vi "DK240 SlitAdjust.vi"(4 "Fente":enum16{"Entrée", "Sortie"}(ring), 5 "error in":errorcluster, 6 "SlitWidth":u16=50 caption="Largeur \nFente (µm)" max=5000 step=1, 7 "MovingRef":refnum<vi>, 8 "Port":refnum<visa-resource-name>="SPECTRO") -> (0 "error out":errorcluster, 2 "Moving":bool caption="Déplacement\nen cours", 3 "Status":u8)   [LabVIEW 2019]
doc: "Ce Vi ajuste la largeur de la fente spécifié à la valeur, en microns, désirée."
uses:
  <vilib>/Utility/error.llb/DialogType.ctl
panel:
  out "Cancel":u8
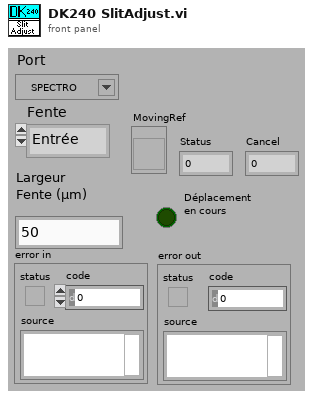
[diagram p1: front panel]
types:
  T1 = enum16{"Commande", "AttendPrêt", "Paramètre", "AttendFin", "Statut", "Fin"}
  T2 = typedef "DialogType.ctl" = u16
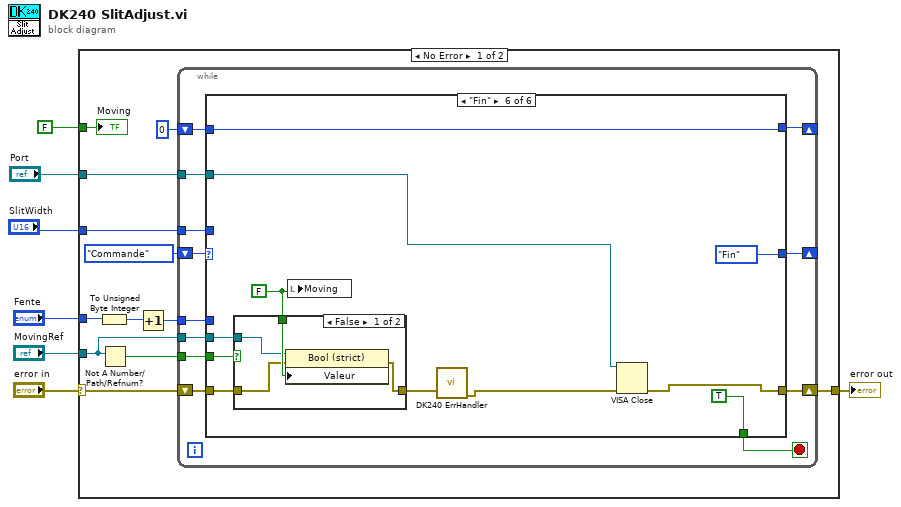
[diagram p0: block diagram]
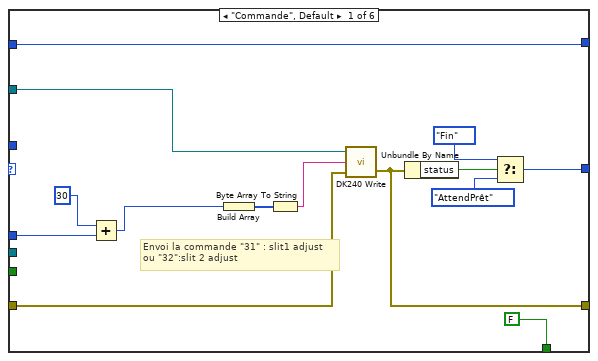
[diagram p2: hidden frame]
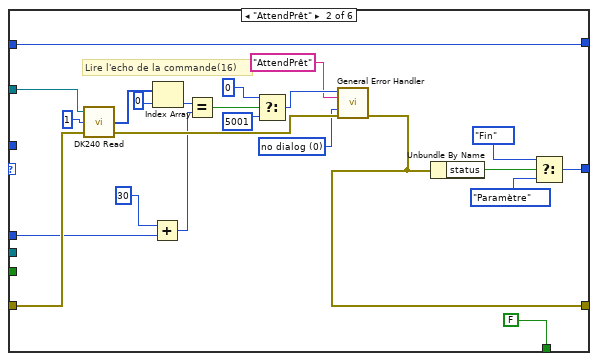
[diagram p3: hidden frame]
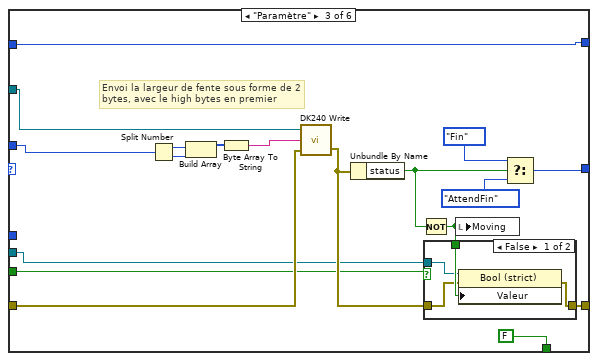
[diagram p4: hidden frame]
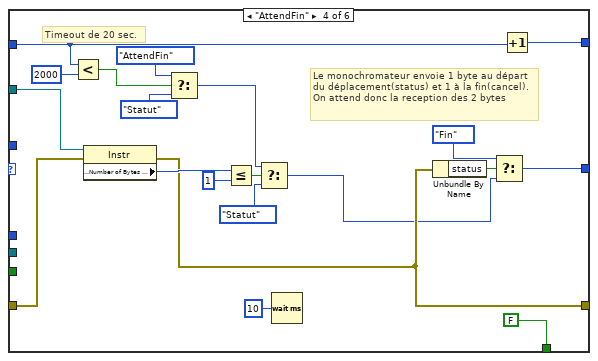
[diagram p6: hidden frame]
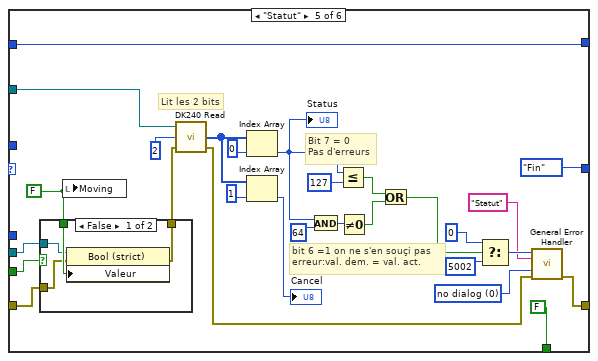
[diagram p7: hidden frame]
diagram:
  n1 = case shown="No Error" "error in" {
    selector: "error in" -> [w15 w161]
    tunnel: "Port" -> [w18 _]
    tunnel: "SlitWidth" -> [w17 _]
    tunnel: [w16 w161] -> w6
    tunnel: FALSE ("Moving") -> [w14 _]
    tunnel: "Fente" -> [w9 _]
    tunnel: "MovingRef" -> [w10 _]
    frame No Error {
      n2 = To Unsigned Byte Integer(number=w9) -> (unsigned 8bit integer=w8:u8)
      n3 = Not A Number/Path/Refnum?(number/path/refnum=w10) -> (NaN/Path/Refnum?=w11:bool)
      n4 = Increment(x=w8) -> (x+1=w13:u8)
      n5 = while {
        shift-right: [w27] -> _
        shift-left: T1."Commande" -> [w31]
        tunnel: w18 -> [w30]
        shift-right: [w28] -> w16
        shift-left: w15 -> [w29]
        tunnel: w17 -> [w26]
        tunnel: w13 -> [w24]
        shift-right: [w23] -> _
        shift-left: 0 -> [w22]
        tunnel: w11 -> [w21]
        tunnel: w10 -> [w20]
        stop <- w25 stop-if-true
        n6 = case shown="\"Fin\"" w31 {
          tunnel: w30 -> [w43 w61 w86 w103 w135 w147]
          tunnel: w29 -> [w42 w60 w85 w111 w114 w152]
          tunnel: [w41 w57 w78 w101 w124 w148] -> w28
          tunnel: [w37 w65 w82 w104 T1."Fin" T1."Fin"] -> w27
          tunnel: w26 -> [_ _ w72 _ _ _]
          tunnel: [FALSE FALSE FALSE FALSE FALSE TRUE] -> w25
          tunnel: w24 -> [w32 w46 _ _ _ _]
          tunnel: [w33 w47 w71 w99 w115 w151] -> w23
          tunnel: w22 -> [w33 w47 w71 w95 w115 w151]
          tunnel: w21 -> [_ _ w70 _ w113 w150]
          tunnel: w20 -> [_ _ w69 _ w112 w149]
          frame "Commande", Default {
            # "Envoi la commande \"31\" : slit1 adjust\nou \"32\":slit 2 adjust"
            n7 = Add(x=u8 30, y=w32) -> (x+y=w34:u8)
            n8 = Build Array(w34) -> (w44:u8[])
            n9 = Byte Array To String(unsigned byte array=w44) -> (string=w45:string)
            n10 = call <userlib>:"DK240 Write.vi"("error in"=w42, "String to write"=w45, "Port"=w43) -> ("error out"=w41:errorcluster)  [unwired: 1 in]
            n11 = Unbundle By Name(w41) -> ("status"=w40:bool)
            n12 = Select(t=T1."Fin", s=w40, f=T1."AttendPrêt") -> (s? t:f=w37:T1)
          }
          frame "AttendPrêt" {
            w51 = T2 0 items=["no dialog", "OK message", "continue or stop message", "OK message + warnings", "continue/stop + warnings"] ("type of dialog (OK msg:1)")
            # "Lire l'echo de la commande(16)"
            n13 = call <userlib>:"DK240 Read.vi"("error in"=w60, "Byte count"=u32 1, "Port"=w61) -> ("error out"=w58:errorcluster, "Received Bytes"=w64:u8[])  [unwired: 1 in]
            n14 = Add(x=u8 30, y=w46) -> (x+y=w48:u8)
            n15 = Index Array(array=w64, index=0) -> (element=w59:u8)
            n16 = Equal?(x=w59, y=w48) -> (x = y?=w56:bool)
            n17 = Select(t=0, s=w56, f=5001 ("t")) -> (s? t:f=w55:i32)
            n18 = call <vilib>:"General Error Handler.vi"("[error code] (0)"=w55, "[error source] (\" \")"="AttendPrêt" ("[error source] (\" \")"), "type of dialog (OK msg:1)"=w51, "error in (no error)"=w58) -> ("error out"=w57:errorcluster)  [unwired: 7 in, 4 out]
            n19 = Unbundle By Name(w57) -> ("status"=w68:bool)
            n20 = Select(t=T1."Fin", s=w68, f=T1."Paramètre") -> (s? t:f=w65:T1)
          }
          frame "Paramètre" {
            # "Envoi la largeur de fente sous forme de 2 bytes, avec le high bytes en premier"
            n21 = Split Number(x=w72) -> (hi(x)=w75:u8, lo(x)=w74:u8)
            n22 = Build Array(w75, w74) -> (w76:u8[])
            n23 = Byte Array To String(unsigned byte array=w76) -> (string=w73:string)
            n24 = call <userlib>:"DK240 Write.vi"("error in"=w85, "String to write"=w73, "Port"=w86) -> ("error out"=w77:errorcluster)  [unwired: 1 in]
            n25 = Unbundle By Name(w77) -> ("status"=w80:bool)
            n26 = Not(x=w80) -> (.not. x?=w79:bool)
            n27 = case shown="False" w70 {
              tunnel: w79 -> [w90 _]
              tunnel: [w89 w91] -> w78
              tunnel: w77 -> [w88 w91]
              tunnel: w69 -> [w87 _]
              frame False {
                n28 = property class="Bool (strict)"(reference=w87, error in=w88, "Valeur"=w90) -> (error out=w89:errorcluster)  [unwired: 1 out]
              }
              frame True {
              }
            }
            n29 = local write "Moving"(w79) -> ()
            n30 = Select(t=T1."Fin", s=w80, f=T1."AttendFin") -> (s? t:f=w82:T1)
          }
          frame "AttendFin" {
            # "Timeout de 20 sec."
            # "Le monochromateur envoie 1 byte au départ du déplacement(status) et 1 à la fin(cancel). On attend donc la reception des 2 bytes"
            n31 = Less?(x=w95, y=2000) -> (x < y?=w93:bool)
            n32 = property class="Instr"(reference=w103, error in=w111) -> (error out=w101:errorcluster, "Serial Settings:Number of Bytes at Serial Port"=w110:u32)  [unwired: 1 out]
            n33 = Select(t=T1."AttendFin", s=w93, f=T1."Statut") -> (s? t:f=w98:T1)
            n34 = Less Or Equal?(x=w110, y=u32 1) -> (x <= y?=w106:bool)
            n35 = Select(t=w98, s=w106, f=T1."Statut") -> (s? t:f=w100:T1)
            n36 = Wait (ms)(milliseconds to wait=u32 10) -> ()  [unwired: 1 out]
            n37 = Unbundle By Name(w101) -> ("status"=w108:bool)
            n38 = Select(t=T1."Fin", s=w108, f=w100) -> (s? t:f=w104:T1)
            n39 = Increment(x=w95) -> (x+1=w99:i32)
          }
          frame "Statut" {
            w129 = T2 0 items=["no dialog", "OK message", "continue or stop message", "OK message + warnings", "continue/stop + warnings"] ("type of dialog (OK msg:1)")
            w117 = FALSE
            # "bit 6 =1 on ne s'en souçi pas \nerreur:val. dem. = val. act."
            # "Bit 7 = 0\nPas d'erreurs"
            # "Lit les 2 bits"
            n40 = case shown="False" w113 {
              tunnel: w117 -> [w143 _]
              tunnel: [w142 w144] -> w116
              tunnel: w114 -> [w141 w144]
              tunnel: w112 -> [w140 _]
              frame False {
                n41 = property class="Bool (strict)"(reference=w140, error in=w141, "Valeur"=w143) -> (error out=w142:errorcluster)  [unwired: 1 out]
              }
              frame True {
              }
            }
            n42 = local write "Moving"(w117) -> ()
            n43 = call <userlib>:"DK240 Read.vi"("error in"=w116, "Byte count"=u32 2, "Port"=w135) -> ("error out"=w128:errorcluster, "Received Bytes"=w139:u8[])  [unwired: 1 in]
            n44 = Index Array(array=w139, index=0) -> (element=w120:u8)
            "Status" <- w120
            n45 = Index Array(array=w139, index=1) -> (element=→"Cancel":u8)
            n46 = And(x=w120, y=u8 64) -> (x .and. y?=w126:u8)
            n47 = Less Or Equal?(x=w120, y=u8 127) -> (x <= y?=w123:bool)
            n48 = Not Equal To 0?(x=w126) -> (x != 0?=w122:bool)
            n49 = Or(x=w123, y=w122) -> (x .or. y?=w121:bool)
            n50 = Select(t=0, s=w121, f=5002 ("t")) -> (s? t:f=w133:i32)
            n51 = call <vilib>:"General Error Handler.vi"("[error code] (0)"=w133, "[error source] (\" \")"="Statut" ("[error source] (\" \")"), "type of dialog (OK msg:1)"=w129, "error in (no error)"=w128) -> ("error out"=w124:errorcluster)  [unwired: 7 in, 4 out]
          }
          frame "Fin" {
            w153 = FALSE
            n52 = case shown="False" w150 {
              tunnel: w153 -> [w159 _]
              tunnel: w152 -> [w158 w160]
              tunnel: [w157 w160] -> w146
              tunnel: w149 -> [w156 _]
              frame False {
                n53 = property class="Bool (strict)"(reference=w156, error in=w158, "Valeur"=w159) -> (error out=w157:errorcluster)  [unwired: 1 out]
              }
              frame True {
              }
            }
            n54 = local write "Moving"(w153) -> ()
            n55 = call <userlib>:"DK240 ErrHandler.vi"("error in"=w146) -> ("error out"=w145:errorcluster)  [unwired: 7 in]
            n56 = VISA Close(VISA resource name=w147, error in (no error)=w145) -> (error out=w148:errorcluster)
          }
        }
      }
      "Moving" <- w14
    }
    frame Error {
    }
  }
  "error out" <- w6
